vi "Set Tps Int.vi"(8 "error in (no error)":errorcluster caption="entrée d'erreur (pas d'erreur)", 11 "UI SA en entrée":refnum<class "UI SmarAct.lvclass">) -> (0 "error out":errorcluster caption="sortie d'erreur", 3 "UI SA en sortie":refnum<class "UI SmarAct.lvclass">)   [LabVIEW 2024, in "UI SmarAct.lvclass"]
uses:
  UI SmarAct.lvclass
  UI SmarAct.lvclass/UI SmarAct.ctl
panel:
  out "d_lambda":dbl=0.44435503366880597
  out "lambda_c":dbl=674.8888701568728
  out "lambda_0":dbl=200.6310762
  out "N":i32=2068
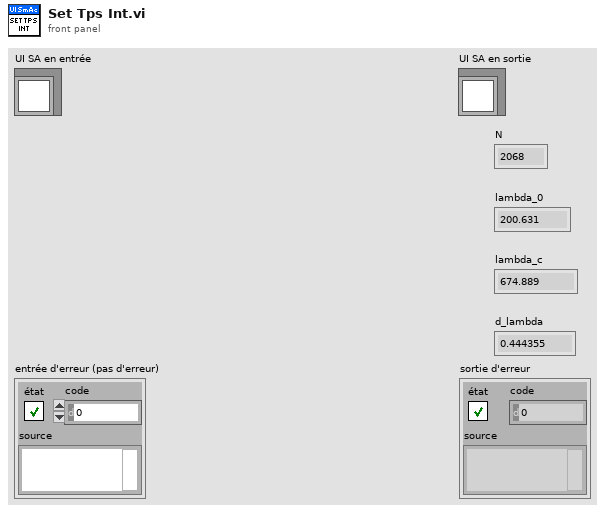
[diagram p1: front panel]
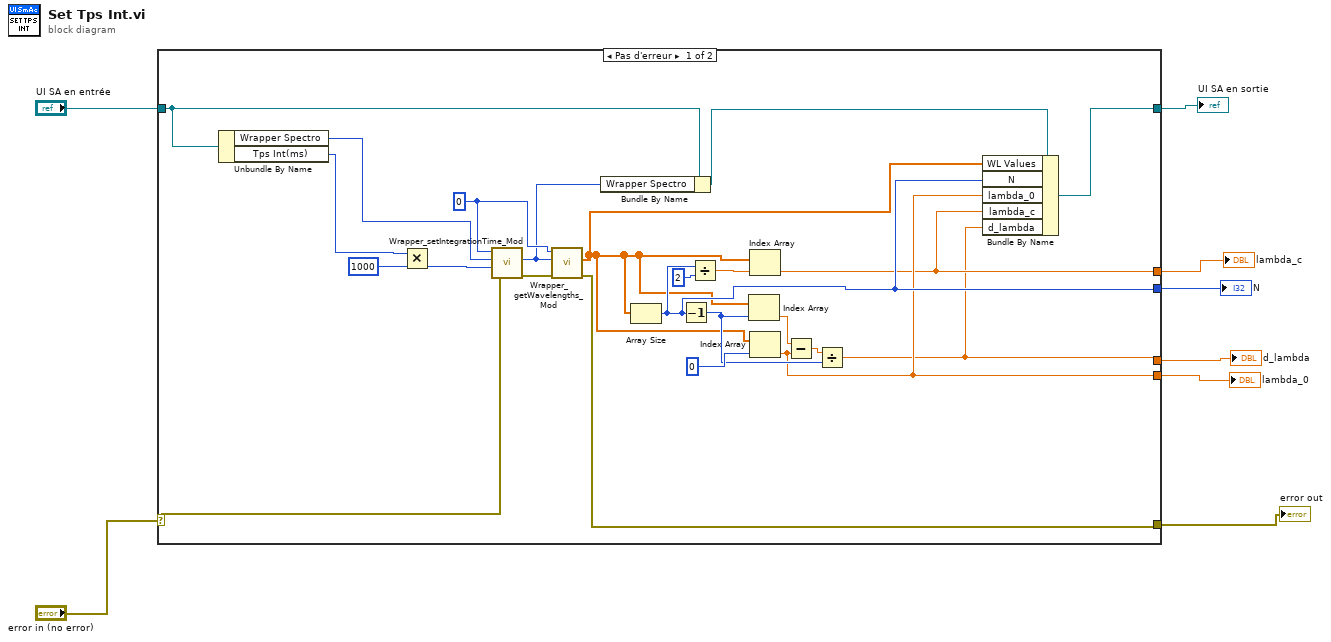
[diagram p0: block diagram]
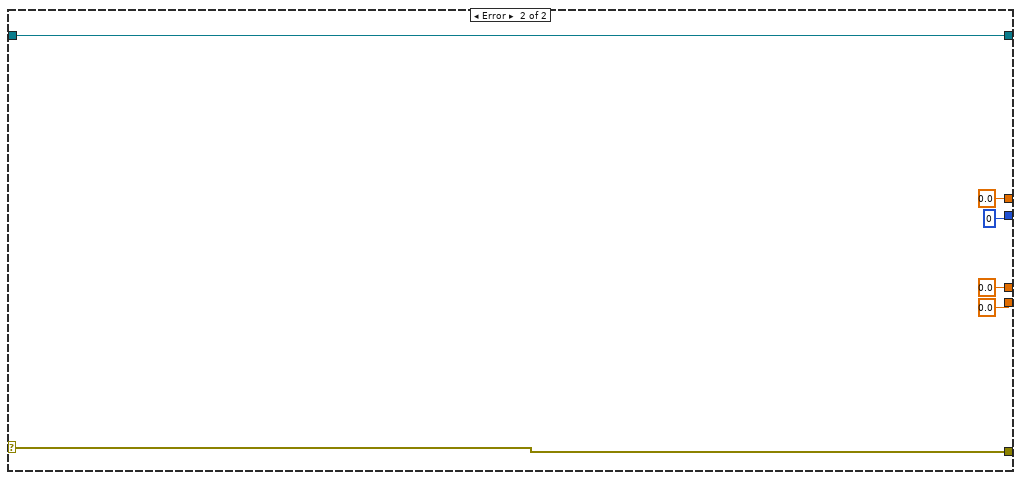
[diagram p2: hidden frame]
diagram:
  n1 = case shown="Pas d'erreur" "error in (no error)" {
    selector: "error in (no error)" -> [w27 w37]
    tunnel: [w24 w37] -> w7
    tunnel: [w14 w36] -> w5
    tunnel: "UI SA en entrée" -> [w29 w36]
    tunnel: [w13 0] -> w4
    tunnel: [w11 0.0] -> w3
    tunnel: [w12 0.0] -> w2
    tunnel: [w10 0.0] -> w1
    frame No Error {
      w23 = 0 ("Index")
      n2 = Unbundle By Name(w29) -> ("Wrapper Spectro"=w28:u32, "Tps Int(ms)"=w26:u32)
      n3 = Multiply(x=w26, y=u32 1000) -> (x*y=w30:u32)
      n4 = call "Wrapper_setIntegrationTime_Mod.vi"("error in (no error)"=w27, "Integration Time"=w30, "Wrapper In"=w28, "Index"=w23) -> ("error out"=w25:errorcluster, "Wrapper Out"=w22:u32)  [unwired: 6 in]
      n5 = call "Wrapper_getWavelengths_Mod.vi"("error in (no error)"=w25, "Wrapper"=w22, "Index"=w23) -> ("error out"=w24:errorcluster, "WL Values"=w9:dbl[])  [unwired: 6 in, 1 out]
      n6 = Bundle By Name(cluster=w29, "Wrapper Spectro"=w22) -> (w15:refnum<class "UI SmarAct.lvclass">)
      n7 = Array Size(array=w9) -> (size(s)=w13:i32)
      n8 = Decrement(x=w13) -> (x-1=w16:i32)
      n9 = Divide(x=w13, y=2) -> (x/y=w19:dbl)
      n10 = Index Array(array=w9, index=w16) -> (element=w18:dbl)
      n11 = Index Array(array=w9, index=w19) -> (element=w11:dbl)
      n12 = Index Array(array=w9, index=0) -> (element=w12:dbl)
      n13 = Subtract(x=w18, y=w12) -> (x-y=w17:dbl)
      n14 = Divide(x=w17, y=w16) -> (x/y=w10:dbl)
      n15 = Bundle By Name(cluster=w15, "WL Values"=w9, "N"=w13, "lambda_0"=w12, "lambda_c"=w11, "d_lambda"=w10) -> (w14:refnum<class "UI SmarAct.lvclass">)
    }
    frame Error {
    }
  }
  "error out" <- w7
  "UI SA en sortie" <- w5
  "N" <- w4
  "lambda_c" <- w3
  "lambda_0" <- w2
  "d_lambda" <- w1
